vi "Bertta_v08.vi"() -> ()   [LabVIEW 2015]
uses:
  <vilib>/Utility/config.llb/Write Key (I32).vi
  <vilib>/Utility/config.llb/Write Key (String).vi
  <vilib>/Utility/config.llb/Write Key (Double).vi
  <vilib>/Utility/Data Type/NI_Data Type.lvlib
  <vilib>/Utility/config.llb/NI_LVConfig.lvlib
panel:
  out "Started:":string
  in  "SHUTDOWN":bool
  in  "OK Button":bool
  in  "Tab Control":T1(tab)
  in  "OK Button 2":bool
  out "Boolean":bool
  in  "User (initials)":string
  in  "Project name":string
  in  "Description":string
  out "Output file":string
  out "PUMP 1":bool
  out "Target amount":dbl
  out "Scale weight":dbl
  out "Amount now":dbl
  out "Flow rate":dbl
  out "Time to target":dbl format="%<%H:%M:%S>t"
  out "Current step":dbl
  out "Target amount":dbl
  out "Amount now":dbl
  out "Tr":dbl
  out "Tj in":dbl
  out "Tj out":dbl
  out "T init":dbl
  out "T set":dbl
  out "Current step":i32
  out "RPM":dbl
  out "Torque 2":dbl
  out "Waveform Chart 5":dynamicdata(graph)
  out "Waveform Chart 6":dynamicdata(graph)
  out "Waveform Chart 7":dynamicdata(graph)
  in  "Tab Control 2":T2(tab)
  out "Waveform Chart 3":dynamicdata(graph)
  out "Waveform Chart 8":dynamicdata(graph)
  out "Waveform Chart 9":dynamicdata(graph)
  out "Table":string[][](table)
  in  "Headers":string[](array[string])=["Flow rate, P1, g/min", "Weight, S1, g", "Amount / step, P1, g", "Step Number, P1", "Total amount, P1, g", "Tj in, C", "Tj out, C", "Tr, C", "RPM", "Torque"]
  out "Boolean 12":bool
  out "Boolean 7":bool
  out "Boolean 6":bool
  out "Boolean 5":bool
  out "Boolean 4":bool
  in  "?":bool
  in  "T manual ctrl":dbl=20.0
  in  "Lauda port":dbl=9.0
  out "Data out":dbl
  in  "Bypass select":enum32{"Tr", "Tj"}(radio)
  in  "Seq":dbl[][](array[numeric])=[[20.0, 45.0, 50.0, 46.0], [46.0, 50.0, 20.0, 51.0], [20.0, 50.0, 3.0, 25.0], [20.0, 20.0, 0.0, 20.0], [20.0, 20.0, 0.0, 20.0], [20.0, 20.0, 1000.0, 20.0]]
  out "T control":dbl
  out "Tr":dbl
  out "Tj in":dbl
  out "Tj out":dbl
  out "DT":dbl
  out "Elapsed":i32
  out "Current step":i32
  in  "PAUSE":bool
  out "Tinit":dbl
  out "Tset":dbl
  out "Time limit":dbl
  out "Waveform Chart":dynamicdata(graph)
  out "Boolean 19":bool
  in  "Reset":bool
  out "Data out":dbl
  in  "Port":i32=10
  in  "Radio Buttons":enum32{"Reglo Digital", "Reglo Analog", "PAM"}(radio)
  out "Speed":dbl
  out "mA":dbl format="%#_2g"
  in  "Port":i32=15
  out "RPM":dbl format="%#_2g"
  out "Boolean 18":bool
  out "Boolean 17":bool
  out "Boolean 16":bool
  out "Boolean 15":bool
  out "Boolean 14":bool
  out "Boolean 13":bool
  out "Boolean 11":bool
  out "Boolean 10":bool
  out "Boolean 9":bool
  out "Boolean 8":bool
  in  "Seq 2":dbl[][](array[numeric])=[[3.0, 3.0, 7.0], [2.0, 2.0, 2.0], [4.0, 2.0, 100.0], [0.0, 0.0, 0.0], [0.0, 0.0, 0.0], [0.0, 0.0, 0.0], [0.0, 0.0, 0.0], [0.0, 0.0, 0.0], [0.0, 0.0, 0.0], [0.0, 0.0, 0.0], [0.0, 1.0, 0.0]]
  in  "?":bool
  out "Flow rate (g/min)":dbl
  out "Time (min)":dbl
  out "Target (g)":dbl
  out "Scale reading":dbl
  out "Step amount now":dbl
  out "Time to target":dbl format="%<%H:%M:%S>t"
  in  "Manual ctrl (g/min)":dbl
  out "Waveform Chart 2":dynamicdata(graph)
  in  "?":bool
  out "Total amount now":dbl
  out "Total time":dbl
  out "Total amount target":dbl
  out "Boolean 20":bool
  in  "Reset 2":bool
  out "RPM":dbl
  out "Torque":dbl
  in  "Set RPM":dbl(slide) scale=0.0..500.0
  out "Waveform Chart 4":dynamicdata(graph)
  in  "?":T3(tab)
  in  "Device port":dbl=13.0
  out "DAQ 9217 (PT100)":errorcluster
  # "PUMP & SCALE 1"
  # "STEP"
  # "TOTAL"
  # "Tinit     >    Tset       min. time       Tfail"
  # "End of sequence"
  # "Grams    /   min"
  # "End of sequence"
  # "Pump configuration"
  # "Scale configuration"
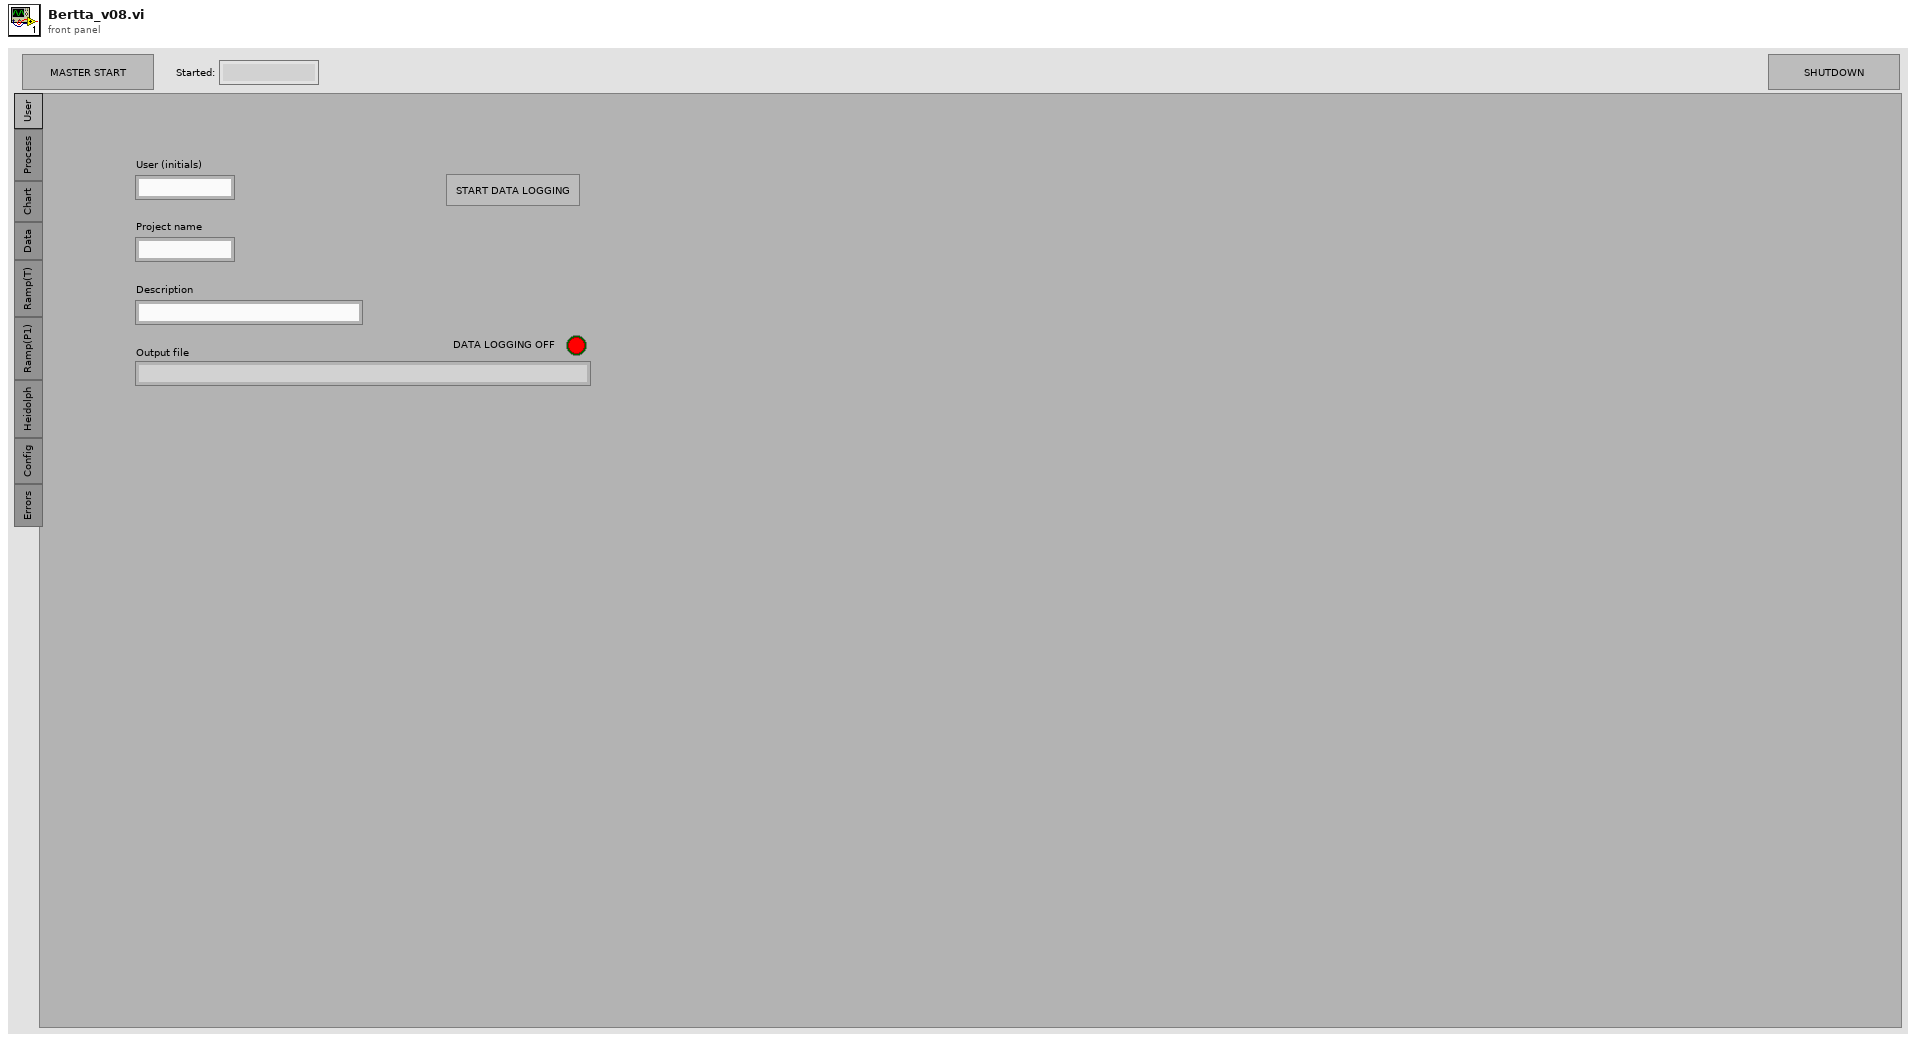
[diagram p1: front panel]
types:
  T1 = enum32{"User", "Process", "Chart", "Data", "Ramp(T)", "Ramp(P1)", "Heidolph", "Config", "Errors"}
  T2 = enum32{"Temperatures", "Scale / Pump 1", "RPM / torque"}
  T3 = enum32{"DB / File", "Lauda", "Heidolph", "Mettler 1", "Mettler 2", "Mettler 3", "Ismatec 1"}
  T4 = typedef "NI_LVConfig.lvlib/Config Data RefNum.ctl" = refnum<k1>
  T5 = typedef "NI_Data Type.lvlib/Data Type.ctl" = enum8{"Invalid Type", "Void", "I8", "I16", "I32", "I64", "U8", "U16", "U32", "U64", "Single Float", "Double Float", "Extended Float", "Single Complex", "Double Complex", "Extended Complex", "Enum U8", "Enum U16", "Enum U32", "Enum U64", "Single Float With Unit", "Double Float With Unit", "Extended Float With Unit", "Single Complex with Unit", "Double Complex with Unit", "Extended Complex with Unit", "Boolean", "String", "Path", "Picture", "Tag", "Array", "Cluster", "Variant", "LV Variant", "Waveform", "Timestamp", "Digital Waveform", "Digital Data", "ExpressData", "Refnum", "External Data", "VI", "Poly VI", "LabVIEW Class Instance", "Fixed Point"}
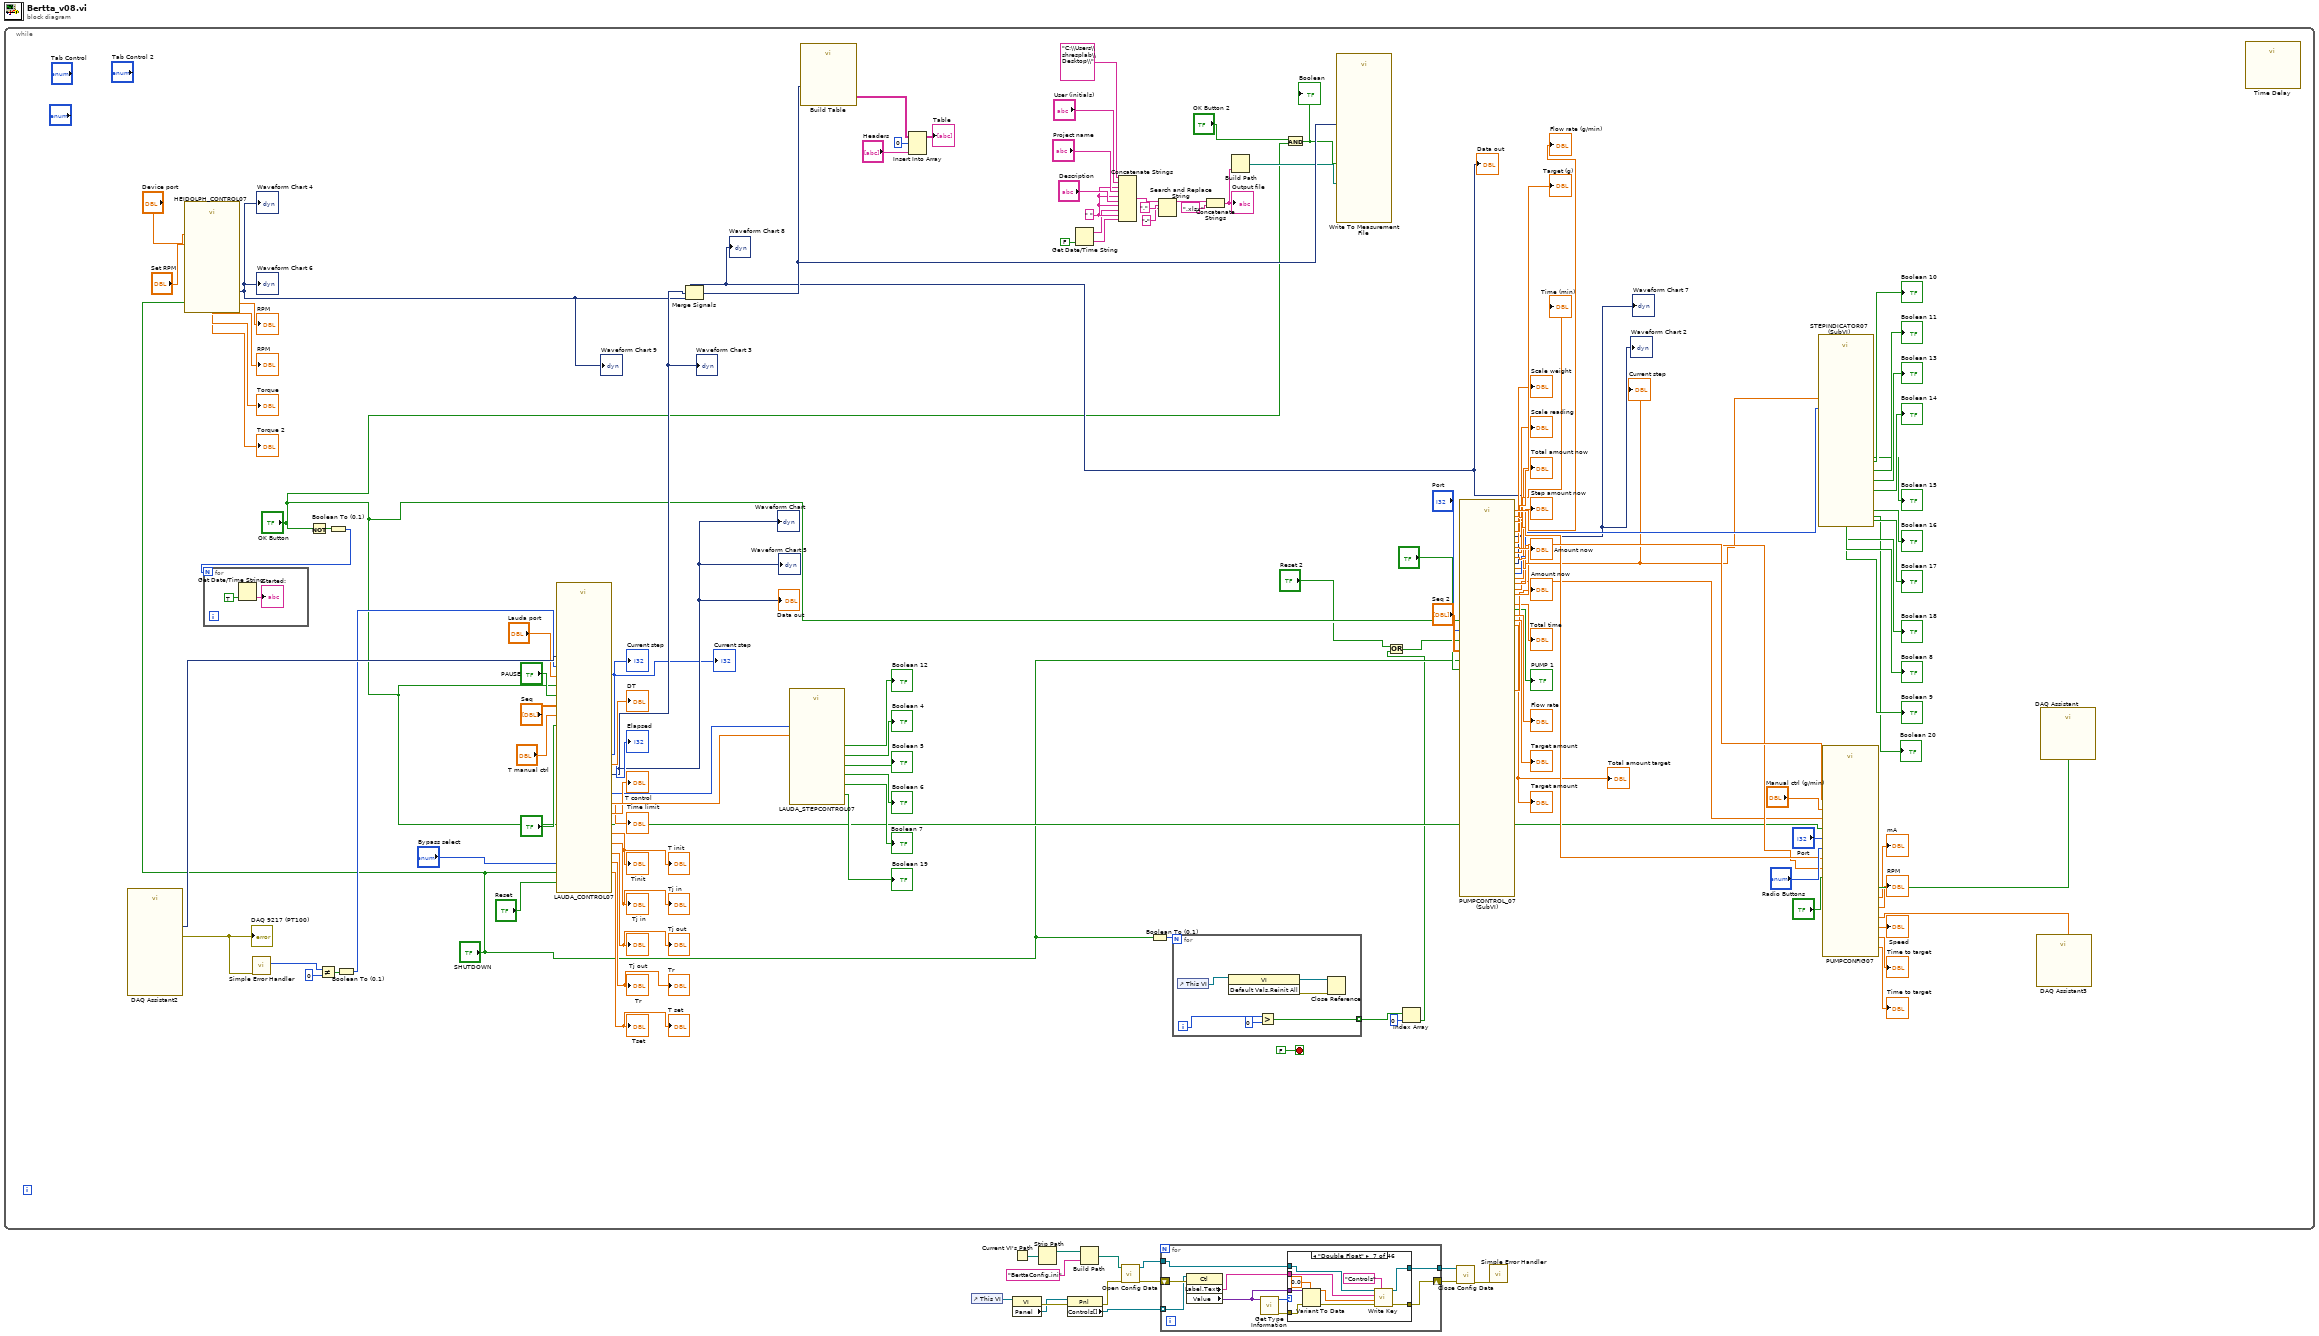
[diagram p0: block diagram]
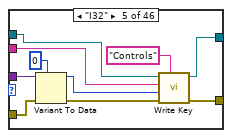
[diagram p6: hidden frame]
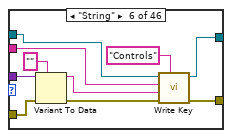
[diagram p7: hidden frame]
diagram:
  n1 = while {
    stop <- FALSE stop-if-true
    w48 = " "
    n2 = call "DAQ Assistant2"() -> ("data"=w119:dynamicdata, "error out"=w57:errorcluster)  [unwired: 17 in, 1 out]
    "DAQ 9217 (PT100)" <- w57
    n3 = call "HEIDOLPH_CONTROL07.vi"("shutdown"="SHUTDOWN", "Set RPM"="Set RPM", "Device port"="Device port") -> ("Dynamic Data"=w63:dynamicdata, "RPM"=→"RPM":dbl, "RPM 2"=→"RPM":dbl, "Torque"=→"Torque":dbl, "Torque 2"=→"Torque 2":dbl)  [unwired: 4 in]
    "Waveform Chart 4" <- w63
    "Waveform Chart 6" <- w63
    "Waveform Chart 9" <- w63
    n4 = call <vilib>:"Simple Error Handler.vi"("error in (no error)"=w57) -> ("code out"=w56:i32)  [unwired: 4 in, 4 out]
    n5 = Not(x="OK Button") -> (.not. x?=w25:bool)
    n6 = Not Equal?(x=w56, y=0) -> (x != y?=w54:bool)
    n7 = Boolean To (0,1)(Boolean=w25) -> (0, 1=w26:i16)
    n8 = for {
      N: w26 -> [_]
      n9 = Get Date/Time String(want seconds? (F)=TRUE) -> (time string=→"Started:":string)  [unwired: 2 in, 1 out]
    }
    n10 = Boolean To (0,1)(Boolean=w54) -> (0, 1=w53:i16)
    n11 = call "LAUDA_CONTROL07.vi"("Master Start"="?", "PAUSE"="PAUSE", "data"=w119, "Seq"="Seq", "Lauda port"="Lauda port", "Tbypass"="T manual ctrl", "Bypass select"="Bypass select", "err"=w53, "Shutdown"="SHUTDOWN", "Bypass"="OK Button", "Reset"="Reset") -> (12:"Tj out"=→"Tj in" →"Tj in":dbl, "DT"=→"DT":dbl, 16:"Tj out"=→"Tj out" →"Tj out":dbl, "Tset"=→"Tset" →"T set":dbl, "Dynamic Data"=w65:dynamicdata, "Time limit"=→"Time limit":dbl, "Numeric"=w31:i16, "Numeric 2"=w125:dbl, "T control"=→"T control":dbl, "Current step"=→"Current step" →"Current step":i32, "Elapsed"=→"Elapsed":i32, "Tr"=→"Tr" →"Tr":dbl, "Tinit"=→"Tinit" →"T init":dbl)  [unwired: 4 in]
    "Waveform Chart 3" <- w65
    "Waveform Chart" <- w65
    "Data out" <- w65
    "Waveform Chart 5" <- w65
    n12 = call "LAUDA_STEPCONTROL07.vi"("Numeric 2"=w125, "Numeric"=w31) -> ("Boolean 13"=→"Boolean 19":bool, "Boolean 6"=→"Boolean 6":bool, "Boolean 5"=→"Boolean 5":bool, "Boolean 4"=→"Boolean 4":bool, "Boolean 7"=→"Boolean 7":bool, "Boolean 12"=→"Boolean 12":bool)  [unwired: 4 in]
    n13 = Get Date/Time String(want seconds? (F)=FALSE) -> (date string=w47:string, time string=w46:string)  [unwired: 2 in]
    n14 = Concatenate Strings("C:\\Users\\shresplab\\Desktop\\", "User (initials)", w48, "Project name", w48, "Description", w48, w47, w48, w46) -> (w43:string)
    n15 = Boolean To (0,1)(Boolean="SHUTDOWN") -> (0, 1=w21:i16)
    n16 = Search and Replace String(input string=w43, search string=".", replace string="-" ("replace string (\"\")")) -> (result string=w40:string)  [unwired: 5 in, 3 out]
    n17 = for {
      N: w21 -> [_]
      tunnel: [w134] -> w17 mode=indexing
      i -> [w136]
      n18 = control-ref of="This VI"() -> (w139:refnum<vi>)
      n19 = invoke class="VI" method="Default Vals.Reinit All"(reference=w139) -> (reference out=w137:refnum<vi>, error out=w138:errorcluster)  [unwired: 2 in, 1 out]
      n20 = Greater?(x=w136, y=0) -> (0:w134:bool)
      n21 = Close Reference(reference=w137, error in (no error)=w138) -> ()  [unwired: 1 out]
    }
    n22 = Concatenate Strings(w40, ".xlsx") -> (w38:string)
    "Output file" <- w38
    n23 = Build Path(name or relative path=w38) -> (appended path=w52:path)  [unwired: 1 in]
    n24 = And(x="OK Button 2", y="OK Button") -> (x .and. y?=w27:bool)
    "Boolean" <- w27
    n25 = Index Array(array=w17, index=0) -> (element=w15:bool)
    n26 = Or(x="Reset 2", y=w15) -> (x .or. y?=w18:bool)
    n27 = call "PUMPCONTROL_07 (SubVI).vi"("Port"="Port", "OK Button"="OK Button", 2:"?", "shutdown"="SHUTDOWN", "Seq in"="Seq 2", "reset"=w18) -> ("Amount now"=→"Amount now":dbl, "Amount now 2"=→"Amount now":dbl, "Flow rate out"=w34:dbl, "Step amount now"=→"Step amount now":dbl, "Total amount now"=→"Total amount now":dbl, "Total time"=→"Total time":dbl, "Numeric 2"=w115:i16, "PUMP 1"=→"PUMP 1":bool, "Numeric"=w110:dbl, "Flow rate"=→"Flow rate":dbl, "Dynamic Data"=w64:dynamicdata, "Target amount"=→"Target amount":dbl, "Time (min) 2"=w116:dbl, "Target amount 2"=→"Total amount target" →"Target amount":dbl, "Scale reading"=→"Scale reading":dbl, "Flow rate (g/min)"=→"Flow rate (g/min)":dbl, "Target (g) 2"=w117:dbl, "Target (g)"=→"Target (g)":dbl, "Time (min)"=→"Time (min)":dbl, "Waveform Chart 2"=→"Waveform Chart 2" →"Waveform Chart 7":dynamicdata, "Scale weight"=→"Scale weight":dbl, "Amount (g)"=w118:dbl)
    "Current step" <- w110
    "Data out" <- w64
    "Waveform Chart 8" <- w64
    n28 = Merge Signals(w64, w65, w63) -> (w66:dynamicdata)
    n29 = call "Build Table"("Signals"=w66) -> ("Table"=w130:string[][])  [unwired: 4 in, 6 out]
    n30 = Insert Into Array(array=w130, index (row)=0, new element="Headers") -> (→"Table":string[][])  [unwired: 1 in]
    n31 = call "Write To Measurement File"("Signals"=w66, "Enable"=w27, "Filename"=w52) -> ()  [unwired: 14 in, 3 out]
    n32 = call "STEPINDICATOR07 (SubVI).vi"("Numeric"=w110, "Numeric 2"=w115) -> ("Boolean 18"=→"Boolean 18":bool, "Boolean 8"=→"Boolean 8":bool, "Boolean 9"=→"Boolean 9":bool, "Boolean 17"=→"Boolean 17":bool, "Boolean 10"=→"Boolean 10":bool, "Boolean 16"=→"Boolean 16":bool, "Boolean 11"=→"Boolean 11":bool, "Boolean 15"=→"Boolean 15":bool, "Boolean 14"=→"Boolean 14":bool, "Boolean 13"=→"Boolean 13":bool, "Boolean 19"=→"Boolean 20":bool)  [unwired: 3 in]
    n33 = call "PUMPCONFIG07.vi"(0:"?", "Radio Buttons"="Radio Buttons", "Bypass (g/min)"="Manual ctrl (g/min)", "Target (g) in"=w117, "Amount (g)"=w118, "Time (min) in"=w116, "Flow rate in"=w34, "OK Button"="OK Button", "Port"="Port") -> ("Time to target 2"=→"Time to target":dbl, "Time to target"=→"Time to target":dbl, "mA"=→"mA":dbl, "signal"=w123:dbl, "Speed"=→"Speed":dbl, "RPM"=→"RPM":dbl, "Array"=w124:bool[])
    n34 = call "DAQ Assistant3"("data"=w123) -> ()  [unwired: 17 in, 2 out]
    n35 = call "DAQ Assistant"("data"=w124) -> ()  [unwired: 17 in, 2 out]
    n36 = call "Time Delay"() -> ()  [unwired: 11 in, 1 out]
  }
  n37 = control-ref of="This VI"() -> (w1:refnum<vi>)
  n38 = property class="VI"(reference=w1) -> (error out=w3:errorcluster, "Panel"=w2:refnum<vi>)  [unwired: 1 in, 1 out]
  n39 = Current VI's Path() -> (path=w5:path)
  n40 = Strip Path(path=w5) -> (stripped path=w6:path)  [unwired: 1 out]
  n41 = property class="Pnl"(reference=w2, error in=w3) -> (error out=w13:errorcluster, "Controls[]"=w4:refnum<vi>[])  [unwired: 1 out]
  n42 = Build Path(base path=w6, name or relative path="BerttaConfig.ini") -> (appended path=w8:path)
  n43 = call <vilib>:"Open Config Data.vi"("error in (no error)"=w13, "configuration file path"=w8) -> ("error out"=w14:errorcluster, "refnum"=w9:T4)  [unwired: 7 in, 1 out]
  n44 = for {
    tunnel: w4 -> [w149] mode=indexing
    tunnel: w9 -> [w145]
    shift-right: [w143] -> w11
    shift-left: w14 -> [w150]
    tunnel: [w144] -> w10
    n45 = property class="Ctl"(reference=w149, error in=w150) -> ("Label.Text"=w146:string, "Value"=w147:variant)  [unwired: 2 out]
    n46 = call <vilib>:"Get Type Information.vi"("Variant"=w147) -> ("error out"=w148:errorcluster, "Type"=w142:T5)  [unwired: 6 in, 3 out]
    n47 = case shown="\"Double Float\"" w142 {
      tunnel: w148 -> [w151 w153 w155 w157 w168 w178 w188 w189 w191 w193 w195 w197 w199 w201 w203 w205 w207 w209 w211 w213 w215 w217 w219 w221 w223 w225 w227 w229 w231 w233 w235 w237 w239 w241 w243 w245 w247 w249 w251 w253 w255 w257 w259 w261 w263 w265]
      tunnel: w147 -> [_ _ _ _ w167 w177 w187 _ _ _ _ _ _ _ _ _ _ _ _ _ _ _ _ _ _ _ _ _ _ _ _ _ _ _ _ _ _ _ _ _ _ _ _ _ _ _]
      tunnel: w146 -> [_ _ _ _ w164 w174 w184 _ _ _ _ _ _ _ _ _ _ _ _ _ _ _ _ _ _ _ _ _ _ _ _ _ _ _ _ _ _ _ _ _ _ _ _ _ _ _]
      tunnel: w145 -> [w152 w154 w156 w158 w163 w173 w183 w190 w192 w194 w196 w198 w200 w202 w204 w206 w208 w210 w212 w214 w216 w218 w220 w222 w224 w226 w228 w230 w232 w234 w236 w238 w240 w242 w244 w246 w248 w250 w252 w254 w256 w258 w260 w262 w264 w266]
      tunnel: [w152 w154 w156 w158 w161 w171 w181 w190 w192 w194 w196 w198 w200 w202 w204 w206 w208 w210 w212 w214 w216 w218 w220 w222 w224 w226 w228 w230 w232 w234 w236 w238 w240 w242 w244 w246 w248 w250 w252 w254 w256 w258 w260 w262 w264 w266] -> w144
      tunnel: [w151 w153 w155 w157 w160 w170 w180 w189 w191 w193 w195 w197 w199 w201 w203 w205 w207 w209 w211 w213 w215 w217 w219 w221 w223 w225 w227 w229 w231 w233 w235 w237 w239 w241 w243 w245 w247 w249 w251 w253 w255 w257 w259 w261 w263 w265] -> w143
      frame "Invalid Type", Default {
      }
      frame "Void" {
      }
      frame "I8" {
      }
      frame "I16" {
      }
      frame "I32" {
        n48 = Variant To Data(error in=w168, type=0, Variant=w167) -> (data=w165:i32, error out=w166:errorcluster)
        n49 = call-poly <vilib>:"Write Key.vi"("section"="Controls", "error in (no error)"=w166, "value"=w165, "key"=w164, "refnum"=w163) -> ("error out"=w160:errorcluster, "refnum out"=w161:T4)  [unwired: 4 in, 1 out]
      }
      frame "String" {
        n50 = Variant To Data(error in=w178, type="", Variant=w177) -> (data=w175:string, error out=w176:errorcluster)
        n51 = call-poly <vilib>:"Write Key.vi"("section"="Controls", "error in (no error)"=w176, "value"=w175, "key"=w174, "refnum"=w173) -> ("error out"=w170:errorcluster, "refnum out"=w171:T4)  [unwired: 4 in, 1 out]
      }
      frame "Double Float" {
        n52 = Variant To Data(error in=w188, type=0.0, Variant=w187) -> (data=w185:dbl, error out=w186:errorcluster)
        n53 = call-poly <vilib>:"Write Key.vi"("section"="Controls", "error in (no error)"=w186, "value"=w185, "key"=w184, "refnum"=w183) -> ("error out"=w180:errorcluster, "refnum out"=w181:T4)  [unwired: 4 in, 1 out]
      }
      frame "I64" {
      }
      frame "U8" {
      }
      frame "U16" {
      }
      frame "U32" {
      }
      frame "U64" {
      }
      frame "Single Float" {
      }
      frame "Extended Float" {
      }
      frame "Single Complex" {
      }
      frame "Double Complex" {
      }
      frame "Extended Complex" {
      }
      frame "Enum U8" {
      }
      frame "Enum U16" {
      }
      frame "Enum U32" {
      }
      frame "Enum U64" {
      }
      frame "Single Float With Unit" {
      }
      frame "Double Float With Unit" {
      }
      frame "Extended Float With Unit" {
      }
      frame "Single Complex with Unit" {
      }
      frame "Double Complex with Unit" {
      }
      frame "Extended Complex with Unit" {
      }
      frame "Boolean" {
      }
      frame "Path" {
      }
      frame "Picture" {
      }
      frame "Tag" {
      }
      frame "Array" {
      }
      frame "Cluster" {
      }
      frame "Variant" {
      }
      frame "LV Variant" {
      }
      frame "Waveform" {
      }
      frame "Timestamp" {
      }
      frame "Digital Waveform" {
      }
      frame "Digital Data" {
      }
      frame "ExpressData" {
      }
      frame "Refnum" {
      }
      frame "External Data" {
      }
      frame "VI" {
      }
      frame "Poly VI" {
      }
      frame "LabVIEW Class Instance" {
      }
      frame "Fixed Point" {
      }
    }
  }
  n54 = call <vilib>:"Close Config Data.vi"("error in (no error)"=w11, "refnum"=w10) -> ("error out"=w12:errorcluster)  [unwired: 8 in, 1 out]
  n55 = call <vilib>:"Simple Error Handler.vi"("error in (no error)"=w12) -> ()  [unwired: 4 in, 5 out]
